vi "Check State Name and Value Uniqueness.vi"(8 "value":i32, 9 "state values":i32[](array[numeric]), 10 "name":string, 11 "state names":string[](array[string])) -> (3 "is unique":bool)   [LabVIEW 2020, in "Routing and Faulting Scripting.lvlib"]
uses:
  Routing and Faulting Scripting.lvlib
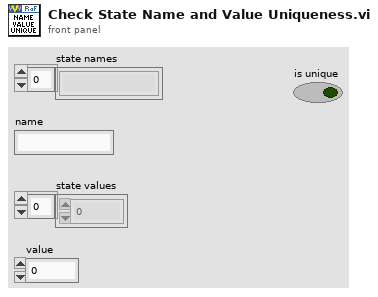
[diagram p1: front panel]
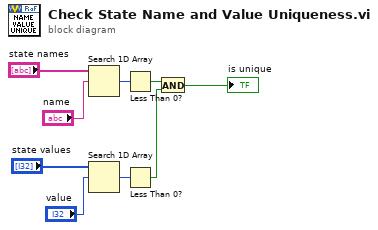
[diagram p0: block diagram]
diagram:
  n1 = Search 1D Array(1D array="state names", element="name") -> (index of element=w4:i32)  [unwired: 1 in]
  n2 = Search 1D Array(1D array="state values", element="value") -> (index of element=w5:i32)  [unwired: 1 in]
  n3 = Less Than 0?(x=w4) -> (x < 0?=w6:bool)
  n4 = Less Than 0?(x=w5) -> (x < 0?=w7:bool)
  n5 = And(x=w6, y=w7) -> (x .and. y?=→"is unique":bool)
